vi "ExecuteCommand.vi"(6 "return immediately":bool, 8 "error in (no error)":errorcluster, 9 "taskId":i32(ring) items=["TLibrary", "T01", "T02", "T03", "T04", "T05", "T06", "T07", "T08", "T09", "T10", "T11", "T12", "T13", "T14", "T15", "T16", "T17", "T18", "T19", "T20", "T21", "T22", "T23", "T24", "T25", "T26", "T27", "T28", "T29", "T30", "T31"], 10 "Command Code":string, 11 "controller in":refnum<k24>) -> (0 "error out":errorcluster, 2 "return value":string, 3 "controller out":refnum<k24>)   [LabVIEW 2021, in "Aerotech.lvlib"]
uses:
  Aerotech.lvlib
  C:/Program Files (x86)/Aerotech/A3200/LabVIEW/2010/Bin/Aerotech.A3200.dll
  Program Files (x86)/Aerotech/A3200/LabVIEW/2010/Bin/Aerotech.A3200.dll
  C:/Program Files (x86)/Aerotech/A3200/LabVIEW/2010/Bin/Aerotech.A3200.LabVIEW.dll
  Program Files (x86)/Aerotech/A3200/LabVIEW/2010/Bin/Aerotech.A3200.LabVIEW.dll
panel:
  in  "Null":refnum<k24>
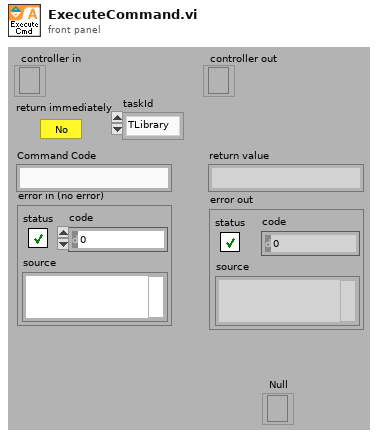
[diagram p1: front panel]
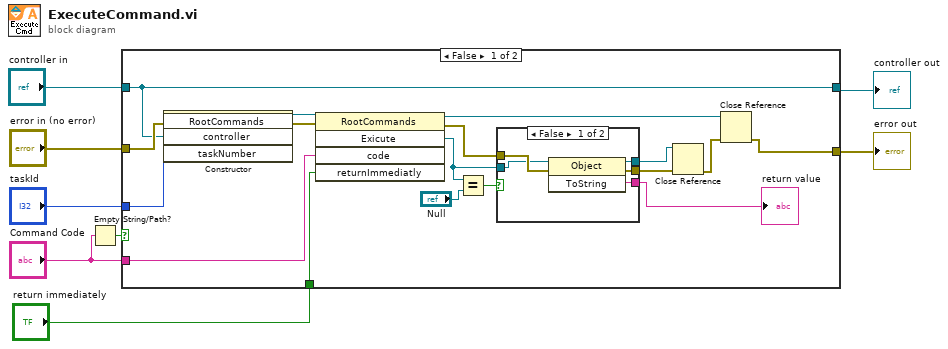
[diagram p0: block diagram]
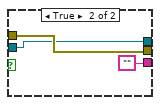
[diagram p2: hidden frame]
diagram:
  n1 = Empty String/Path?(string/path="Command Code") -> (empty?=w3:bool)
  n2 = case shown="False" w3 {
    tunnel: [w11 w34] -> w8
    tunnel: "error in (no error)" -> [w24 w34]
    tunnel: "controller in" -> [w20 w35]
    tunnel: "Command Code" -> [w22 _]
    tunnel: "taskId" -> [w21 _]
    tunnel: [w20 w35] -> w4
    tunnel: "return immediately" -> [w9 _]
    frame False {
      n3 = constructor class="RootCommands"(error in=w24, "controller"=w20, "taskNumber"=w21) -> (reference out=w25:refnum<k24>, error out=w23:errorcluster)  [unwired: 2 in, 3 out]
      n4 = invoke class="RootCommands" method="Exicute"(reference=w25, error in=w23, "code"=w22, "returnImmediatly"=w9) -> (reference out=w13:refnum<k24>, error out=w12:errorcluster, "Exicute"=w10:refnum<k24>)  [unwired: 1 in, 2 out]
      n5 = Equal?(x=w10, y="Null") -> (x = y?=w18:bool)
      n6 = case shown="False" w18 {
        tunnel: w12 -> [w30 w33]
        tunnel: [w29 w33] -> w15
        tunnel: w10 -> [w28 w31]
        tunnel: [w27 ""] -> w19
        tunnel: [w26 w31] -> w14
        frame False {
          n7 = invoke class="Object" method="ToString"(reference=w28, error in=w30) -> (reference out=w26:refnum<k24>, error out=w29:errorcluster, "ToString"=w27:string)  [unwired: 1 in]
        }
        frame True {
        }
      }
      "return value" <- w19
      n8 = Close Reference(reference=w14, error in (no error)=w15) -> (error out=w16:errorcluster)
      n9 = Close Reference(reference=w13, error in (no error)=w16) -> (error out=w11:errorcluster)
    }
    frame True {
    }
  }
  "error out" <- w8
  "controller out" <- w4
